vi "Main.vi"(11 "TestApplication in":refnum<class "TestApplication.lvclass">) -> (3 "TestApplication out":refnum<class "TestApplication.lvclass">)   [LabVIEW 2022 SP3, in "Demo.lvlib" / "TestApplication.lvclass"]
uses:
  TestApplication.lvclass
  TestApplication.lvclass/TestApplication.ctl
  Errors/E55555/E55555.lvclass
  Error/Error/Error.lvclass
  Errors/E11111/E11111.lvclass
  <vilib>/measure/NI_MABase.lvlib
panel:
  out "ErrorCounter":i32
  out "last error":errorcluster
  in  "BtnNoError":bool
  out "error out":errorcluster
  in  "BtnE11111":bool
  in  "BtnGenericError":bool
  out "E55555":bool
  in  "BtnStandardError":bool
  in  "BtnE55555":bool
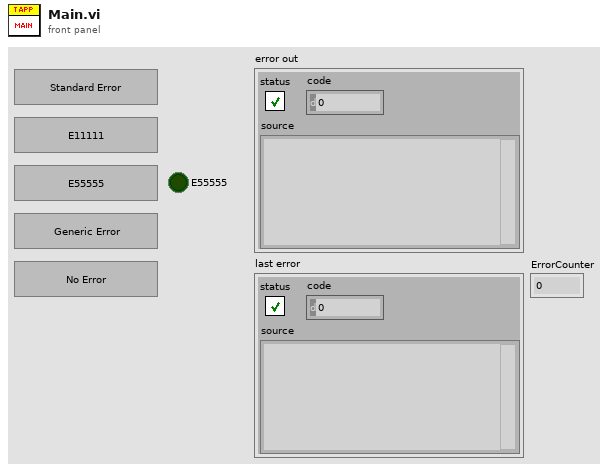
[diagram p1: front panel]
types:
  T1 = typedef "Demo.lvlib/TestApplication.lvclass/_Events.ctl" = cluster{"ToggleLed":refnum<user-event>}
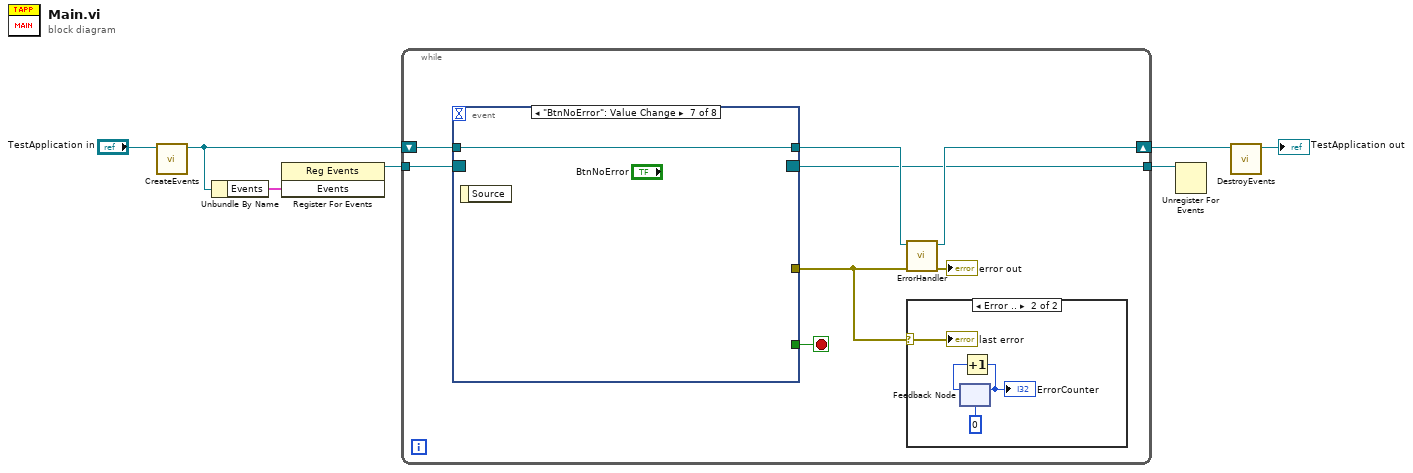
[diagram p0: block diagram]
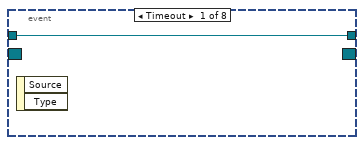
[diagram p3: hidden frame]
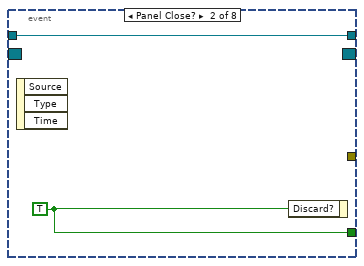
[diagram p4: hidden frame]
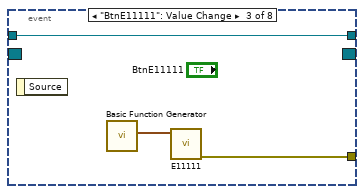
[diagram p5: hidden frame]
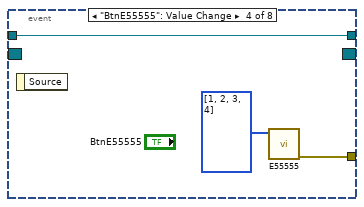
[diagram p6: hidden frame]
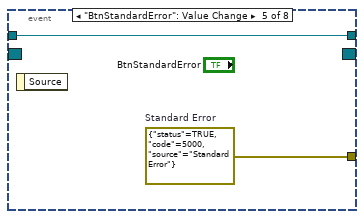
[diagram p7: hidden frame]
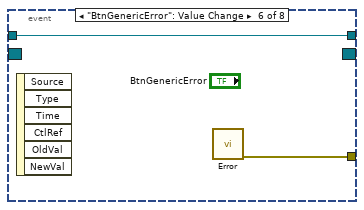
[diagram p8: hidden frame]
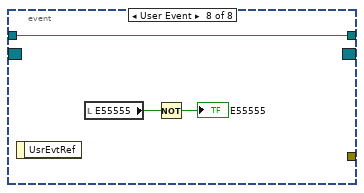
[diagram p9: hidden frame]
diagram:
  n1 = call "CreateEvents.vi"("TestApplication in"="TestApplication in") -> ("TestApplication out"=w5:refnum<class "TestApplication.lvclass">)  [unwired: 9 in, 1 out]
  n2 = Unbundle By Name(w5) -> ("Events"=w4:T1)
  n3 = register-events(w4) -> (reference out=w7:refnum<event-registration>)  [unwired: 2 in, 1 out]
  n4 = while {
    shift-right: [w13] -> w3
    shift-left: w5 -> [w14]
    tunnel: w7 -> [w11]
    tunnel: [w10] -> w1
    stop <- w15 stop-if-true
    n5 = event shown="[6] \"BtnNoError\": Value Change" {
      selector: w11 -> [_ _ _ _ _ _ _ _]
      dyn-events: [_ _ _ _ _ _ _ _] -> w10
      timeout: _ -> [_ _ _ _ _ _ _ _]
      tunnel: [_ w22 _ _ _ _ _ _] -> w15
      tunnel: [_ _ w24 w26 w29 w31 _ _] -> w8
      tunnel: w14 -> [w20 w21 w25 w28 w30 w32 w33 w36]
      tunnel: [w20 w21 w25 w28 w30 w32 w33 w36] -> w12
      event Timeout {
        n6 = event-data() -> ()  [unwired: 1 in, 2 out]
      }
      event Panel Close? {
        w22 = TRUE ("Discard?")
        n7 = event-data() -> ()  [unwired: 1 in, 3 out]
        n8 = event-data("Discard?"=w22) -> ()  [unwired: 1 in, 1 out]
      }
      event "BtnE11111": Value Change {
        n9 = event-data() -> ()  [unwired: 1 in, 1 out]
        n10 = call <vilib>:"Basic Function Generator.vi"() -> ("signal out"=w23:waveform(dbl))  [unwired: 9 in, 2 out]
        n11 = call "E11111.vi"("Signal"=w23) -> ("error out"=w24:errorcluster)  [unwired: 10 in]
      }
      event "BtnE55555": Value Change {
        n12 = event-data() -> ()  [unwired: 1 in, 1 out]
        n13 = call "E55555.vi"("Data"=i32[] [1, 2, 3, 4]) -> ("error out"=w26:errorcluster)  [unwired: 10 in]
      }
      event "BtnStandardError": Value Change {
        w29 = errorcluster {"status"=TRUE, "code"=5000, "source"="Standard Error"}  # Standard Error
        n14 = event-data() -> ()  [unwired: 1 in, 1 out]
      }
      event "BtnGenericError": Value Change {
        n15 = event-data() -> ()  [unwired: 1 in, 6 out]
        n16 = call "Error.vi"() -> ("error out"=w31:errorcluster)  [unwired: 11 in]
      }
      event "BtnNoError": Value Change {
        n17 = event-data() -> ()  [unwired: 1 in, 1 out]
      }
      event User Event {
        n18 = event-data() -> ()  [unwired: 1 in, 1 out]
        n19 = local read "E55555"() -> (w35:bool)
        n20 = Not(x=w35) -> (.not. x?=→"E55555":bool)
      }
    }
    n21 = call-dynamic "ErrorHandler.vi"("error in (no error)"=w8, "TestApplication in"=w12) -> ("error out"=→"error out":errorcluster, "TestApplication out"=w13:refnum<class "TestApplication.lvclass">)  [unwired: 8 in]
    n22 = case shown="Error .." w8 {
      selector: w8 -> [_ w19]
      frame No Error {
      }
      frame Error {
        n23 = feedback #1(0) -> (w17:i32)
        n24 = Increment(x=w17) -> (x+1=w16:i32)
        "ErrorCounter" <- w16
        n25 = feedback-in #1(w16) -> ()
        "last error" <- w19
      }
    }
  }
  n26 = Unregister For Events(event registration refnum=w1) -> ()  [unwired: 1 in, 1 out]
  n27 = call "DestroyEvents.vi"("TestApplication in"=w3) -> ("TestApplication out"=→"TestApplication out":refnum<class "TestApplication.lvclass">)  [unwired: 9 in, 1 out]
